vi "Stop Core.vi"(10 "final error code":i32, 11 "Configurator Actor:Configuration UI Actor in":refnum<class "Configuration UI Actor.lvclass">) -> (3 "Configurator Actor:Configuration UI Actor out":refnum<class "Configuration UI Actor.lvclass">)   [LabVIEW 2023, in "Configuration UI Actor.lvlib" / "Configuration UI Actor.lvclass"]
doc: "(<B>Filename</B>: Actor Framework.lvlib:Actor.lvclass:Stop Core.vi)\n\nDefines what the actor does before it stops. Use the <B>final error code</B> input to determine whether the actor shut down in response to an error.\n\nBy default, this method does nothing. A descendant class may override it to define behavior, such as shutting down any processes the actor initiated in its override of the Actor Core method."
uses:
  Configuration UI Actor.lvclass
  <vilib>/MGI/Panel Manager/Panel Actor/Panel Actor/Panel Actor.lvclass
  Configuration UI Actor.lvclass/Configuration UI Actor.ctl
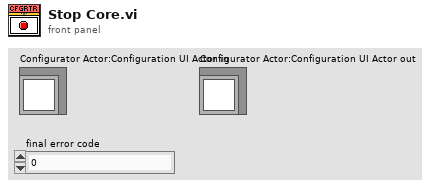
[diagram p1: front panel]
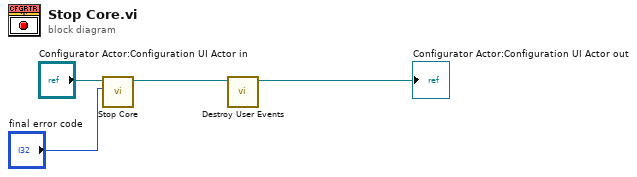
[diagram p0: block diagram]
diagram:
  n1 = call-parent "Stop Core.vi"("final error code"="final error code", "Actor in"="Configurator Actor:Configuration UI Actor in") -> ("Actor out"=w2:refnum<class "Configuration UI Actor.lvclass">)  [unwired: 9 in]
  n2 = call "Destroy User Events.vi"("Configurator Actor:Configuration UI Actor in"=w2) -> ("Configurator Actor:Configuration UI Actor out"=→"Configurator Actor:Configuration UI Actor out":refnum<class "Configuration UI Actor.lvclass">)  [unwired: 10 in]
